vi "创建路径 (子VI).vi"(11 "文件路径（基路径）":path) -> (2 "表格实际路径":path, 3 "appended path":path)   [LabVIEW 2013]
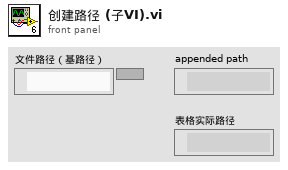
[diagram p1: front panel]
types:
  T1 = enum16{"open", "replace", "create", "open or create", "replace or create", "replace or create with confirmation"}
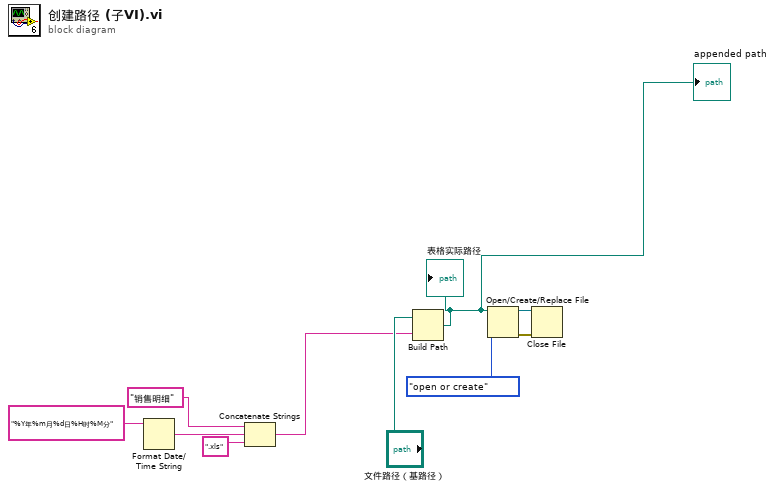
[diagram p0: block diagram]
diagram:
  n1 = Format Date/Time String(time format string (%c)="%Y年%m月%d日%H时%M分") -> (date/time string=w4:string)  [unwired: 2 in]
  n2 = Concatenate Strings("销售明细" ("string"), w4, ".xls" ("string")) -> (w8:string)
  n3 = Build Path(base path="文件路径（基路径）", name or relative path=w8) -> (appended path=w9:path)
  "表格实际路径" <- w9
  "appended path" <- w9
  n4 = Open/Create/Replace File(file path (use dialog)=w9, operation (0:open)=T1."open or create" ("操作(0:open)")) -> (refnum out=w6:refnum<file>, error out=w5:errorcluster)  [unwired: 1 in, 4 out]
  n5 = Close File(refnum=w6, error in=w5) -> ()  [unwired: 2 out]
